vi "Go To Target.vi"(1 "Known Inputs":T9={"Robot Drive Ref"={"DevStatus"={"status"=FALSE, "code"=0, "source"=""}, "Motors[]"=[], "Square Inputs"=FALSE, "Max Output"=1.0}, "Object Position"=0, "Current Disance"=0}, 2 "Settings":T10) -> ()   [LabVIEW 2015]
uses:
  <vilib>/Rock Robotics/WPI/RobotDrive/WPI_RobotDriveDevRef.ctl
  <vilib>/Rock Robotics/WPI/MotorControl/WPI_MotorControlDeviceRef.ctl
  <vilib>/Rock Robotics/WPI/MotorControl/WPI_MotorControlType.ctl
  <vilib>/Rock Robotics/SystemInterfaces/DIO/FPGA_DIOPWMChannel.ctl
  <vilib>/Rock Robotics/WPI/PWM/WPI_PWMDeadband.ctl
  <vilib>/Rock Robotics/WPI/CAN/Jaguar/SubVIs/WPI_CANJaguar_ControlMode.ctl
  <vilib>/Rock Robotics/WPI/CAN/TalonSRX/WPI_CANTalonSRX_APIControlMode.ctl
  <vilib>/Rock Robotics/WPI/RobotDrive/WPI_RobotDriveMecanumDrive_Cartesian.vi
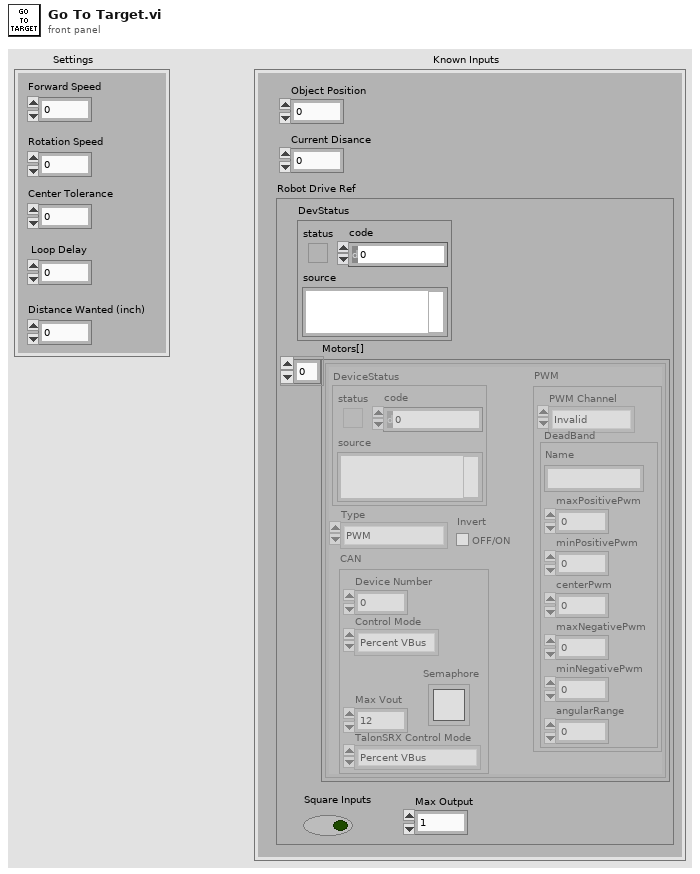
[diagram p1: front panel]
types:
  T1 = typedef "WPI_RobotDriveDevRef.ctl" = cluster{"DevStatus":errorcluster, "Motors[]":T2[], "Square Inputs":bool, "Max Output":dbl}
  T2 = typedef "WPI_MotorControlDeviceRef.ctl" = cluster{"DeviceStatus":errorcluster, "Type":T3, "PWM":cluster{"PWM Channel":T4, "DeadBand":T5}, "CAN":cluster{"Device Number":u8, "Control Mode":T6, "Semaphore":T7, "Max Vout":dbl, "TalonSRX Control Mode":T8}, "Invert":bool}
  T3 = typedef "WPI_MotorControlType.ctl" = enum16{"PWM", "CAN", "CANTalonSRX"}
  T4 = typedef "FPGA_DIOPWMChannel.ctl" = enum8{"PWM 0", "PWM 1", "PWM 2", "PWM 3", "PWM 4", "PWM 5", "PWM 6", "PWM 7", "PWM 8", "PWM 9", "PWM MXP 0", "PWM MXP 1", "PWM MXP 2", "PWM MXP 3", "PWM MXP 4", "PWM MXP 5", "PWM MXP 6", "PWM MXP 7", "PWM MXP 8", "PWM MXP 9", "Invalid"}
  T5 = typedef "WPI_PWMDeadband.ctl" = cluster{"Name":string, "maxPositivePwm":i32, "minPositivePwm":i32, "centerPwm":i32, "maxNegativePwm":i32, "minNegativePwm":i32, "angularRange":u16}
  T6 = typedef "WPI_CANJaguar_ControlMode.ctl" = enum8{"Percent VBus", "Current", "Speed", "Position", "Voltage"}
  T7 = typedef "Semaphore RefNum" = refnum<k1>
  T8 = typedef "WPI_CANTalonSRX_APIControlMode.ctl" = enum8{"Percent VBus", "Speed", "Position", "Slave", "Unchanged / Invalid", "Voltage Compensation", "Current", "Motion Profile"}
  T9 = cluster{"Robot Drive Ref":T1, "Object Position":i32, "Current Disance":i32}
  T10 = cluster{"Forward Speed":dbl, "Rotation Speed":dbl, "Center Tolerance":i32, "Loop Delay":u32, "Distance Wanted (inch)":i32}
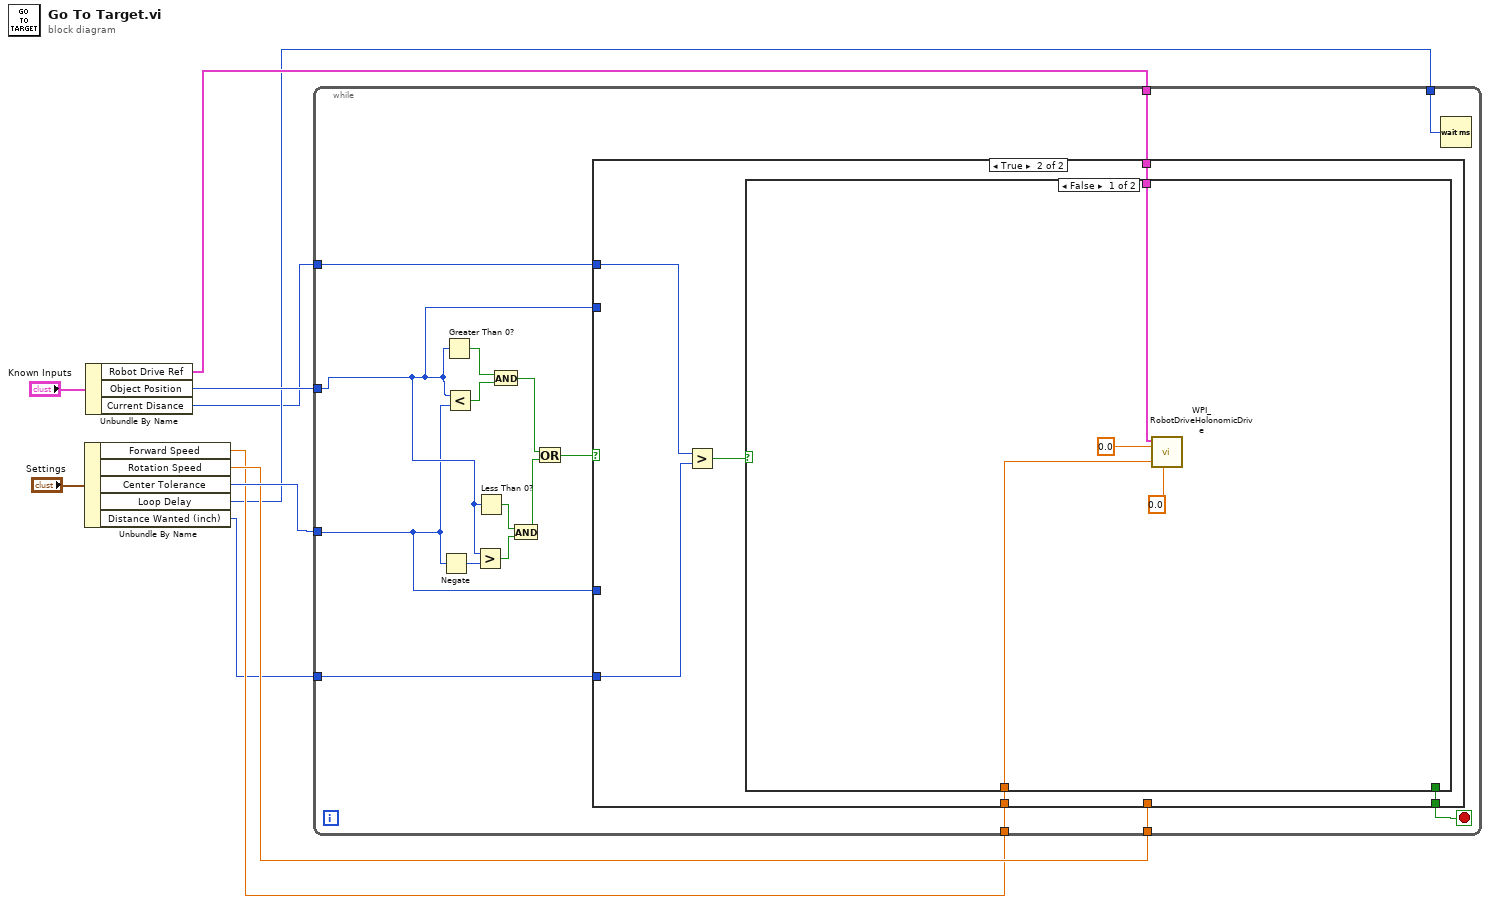
[diagram p0: block diagram]
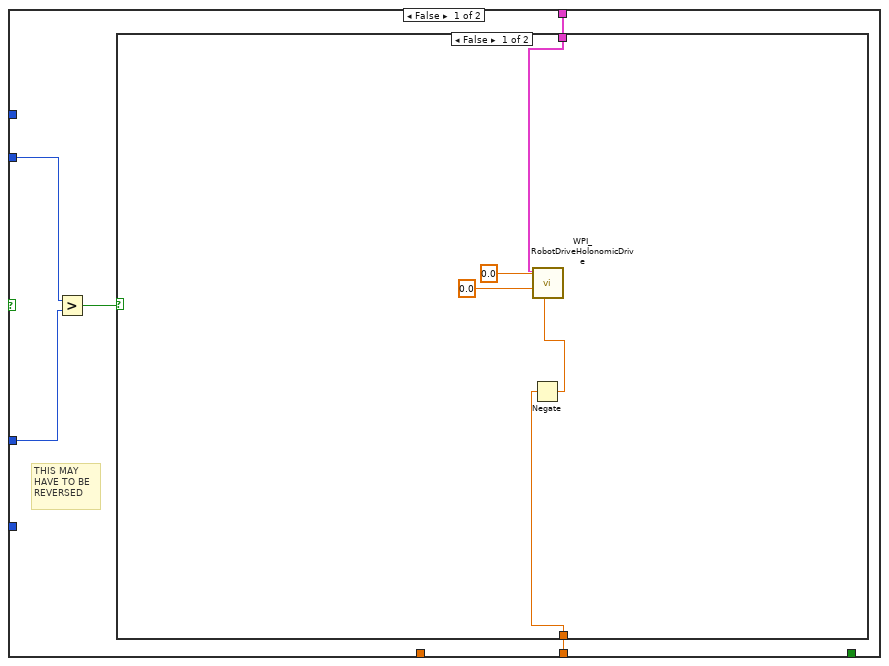
[diagram p2: hidden frame]
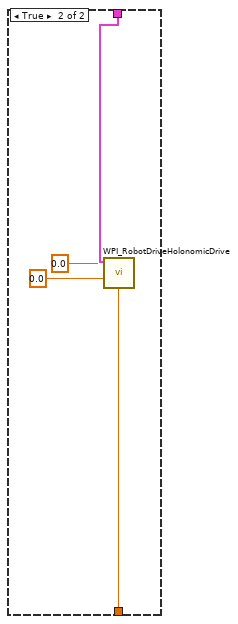
[diagram p3: hidden frame]
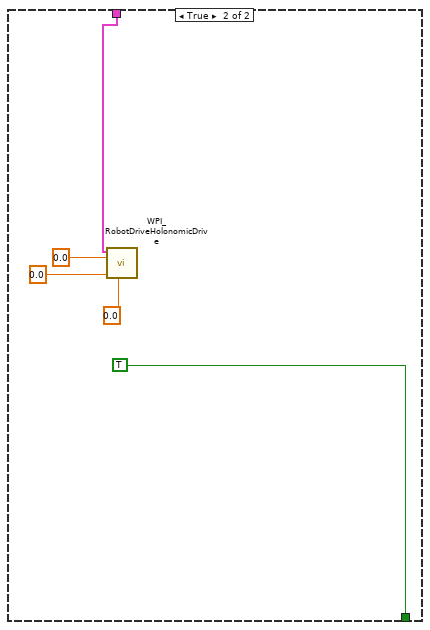
[diagram p4: hidden frame]
diagram:
  n1 = Unbundle By Name("Settings") -> ("Forward Speed"=w4:dbl, "Rotation Speed"=w5:dbl, "Center Tolerance"=w7:i32, "Loop Delay"=w3:u32, "Distance Wanted (inch)"=w1:i32)
  n2 = Unbundle By Name("Known Inputs") -> ("Robot Drive Ref"=w6:T1, "Object Position"=w8:i32, "Current Disance"=w2:i32)
  n3 = while {
    tunnel: w6 -> [w20]
    tunnel: w5 -> [w17]
    tunnel: w8 -> [w16]
    tunnel: w7 -> [w15]
    tunnel: w4 -> [w14]
    tunnel: w3 -> [w13]
    tunnel: w2 -> [w12]
    tunnel: w1 -> [w11]
    stop <- w21 stop-if-true
    n4 = Negate(x=w15) -> (-x=w24:i32)
    n5 = Greater Than 0?(x=w16) -> (x > 0?=w27:bool)
    n6 = Less?(x=w16, y=w15) -> (x < y?=w26:bool)
    n7 = Greater?(x=w16, y=w24) -> (0:w23:bool)
    n8 = Less Than 0?(x=w16) -> (x < 0?=w22:bool)
    n9 = And(x=w27, y=w26) -> (x .and. y?=w19:bool)
    n10 = And(x=w22, y=w23) -> (x .and. y?=w18:bool)
    n11 = Or(x=w19, y=w18) -> (x .or. y?=w25:bool)
    n12 = case shown="True" w25 {
      tunnel: [_ w46] -> w21
      tunnel: w20 -> [w29 w45]
      tunnel: w15 -> [w31 _]
      tunnel: w16 -> [w32 _]
      tunnel: w17 -> [w28 _]
      tunnel: w14 -> [_ w44]
      tunnel: w12 -> [_ w43]
      tunnel: w11 -> [_ w42]
      frame False {
        # "THIS MAY \nHAVE TO BE\nREVERSED"
        n13 = Greater?(x=w32, y=w31) -> (0:w30:bool)
        n14 = case shown="False" w30 {
          tunnel: w29 -> [w35 w41]
          tunnel: w28 -> [w33 w38]
          frame False {
            n15 = Negate(x=w33) -> (-x=w34:dbl)
            n16 = call-poly <vilib>:"WPI_RobotDriveHolonomicDrive.vi"("Rotation"=w34, "Y"=0.0, "X"=0.0, "RobotDriveDevRef"=w35) -> ()  [unwired: 5 in, 3 out]
          }
          frame True {
            n17 = call-poly <vilib>:"WPI_RobotDriveHolonomicDrive.vi"("Rotation"=w38, "Y"=0.0, "X"=0.0, "RobotDriveDevRef"=w41) -> ()  [unwired: 5 in, 3 out]
          }
        }
      }
      frame True {
        n18 = Greater?(x=w43, y=w42) -> (0:w47:bool)
        n19 = case shown="False" w47 {
          tunnel: [_ TRUE] -> w46
          tunnel: w45 -> [w49 w52]
          tunnel: w44 -> [w48 _]
          frame False {
            n20 = call-poly <vilib>:"WPI_RobotDriveHolonomicDrive.vi"("Rotation"=0.0, "Y"=w48, "X"=0.0, "RobotDriveDevRef"=w49) -> ()  [unwired: 5 in, 3 out]
          }
          frame True {
            n21 = call-poly <vilib>:"WPI_RobotDriveHolonomicDrive.vi"("Rotation"=0.0, "Y"=0.0, "X"=0.0, "RobotDriveDevRef"=w52) -> ()  [unwired: 5 in, 3 out]
          }
        }
      }
    }
    n22 = Wait (ms)(milliseconds to wait=w13) -> ()  [unwired: 1 out]
  }
